vi "Image Data to Byte Array.vi"(8 "错误输入（无错误）":errorcluster, 10 "Byte Array Format":enum32{"PNG", "JPEG", "EMF"}(ring), 11 "Image Data":T1) -> (0 "错误输出":errorcluster, 3 "Image Data To Byte Array":u8[](array[numeric]))   [LabVIEW 2012, in "Application.lvlib"]
uses:
  Application.lvlib
  <vilib>/picture/picture.llb/imagedata.ctl
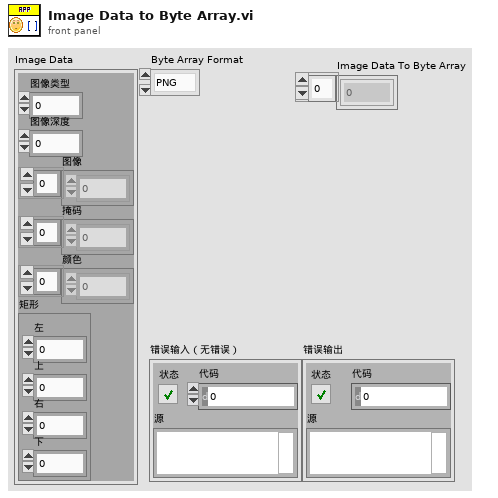
[diagram p1: front panel]
types:
  T1 = typedef "imagedata.ctl" = cluster{"image type":i32, "image depth":i32, "image":u8[], "mask":u8[], "colors":u32[], "Rectangle":cluster{"left":i16, "top":i16, "right":i16, "bottom":i16}}
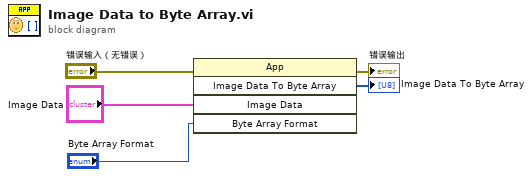
[diagram p0: block diagram]
diagram:
  n1 = invoke class="App" method="Image Data To Byte Array"(error in="错误输入（无错误）", "Image Data"="Image Data", "Byte Array Format"="Byte Array Format") -> (error out=→"错误输出":errorcluster, "Image Data To Byte Array"=→"Image Data To Byte Array":u8[])  [unwired: 2 in, 3 out]
